vi "Analyse.vi"(0 "object in":refnum<class "StateReverse.lvclass">, 1 "NextState":string, 2 "StateAction":T1, 3 "NextStateComments":string, 5 "error in (no error)":errorcluster) -> (15 "StateTransitions":cluster{"StateTransitions":string[]}[](array[cluster]), 16 "CommentsTransitions":cluster{"StateTransitions":string[]}[](array[cluster]), 19 "error out":errorcluster)   [LabVIEW 2012, in "StateReverse.lvclass"]
uses:
  <resource>/Framework/Providers/Open_GDS/UML/StateReverse_class/StateReverse.lvclass
  <resource>/Framework/Providers/Open_GDS/UML/StateReverse_class/StateAction.ctl
  <resource>/Framework/Providers/Open_GDS/UML/ReversedEngineering/ReversedEngineering StateMachineStateInfo.ctl
  <resource>/Framework/Providers/Open_GDS/UML/StateReverse_class/StateReverse.lvclass/StateReverse.ctl
  <resource>/Framework/Providers/Open_GDS/UML/UMLEditor/UMLEditor BusyDialogAction.ctl
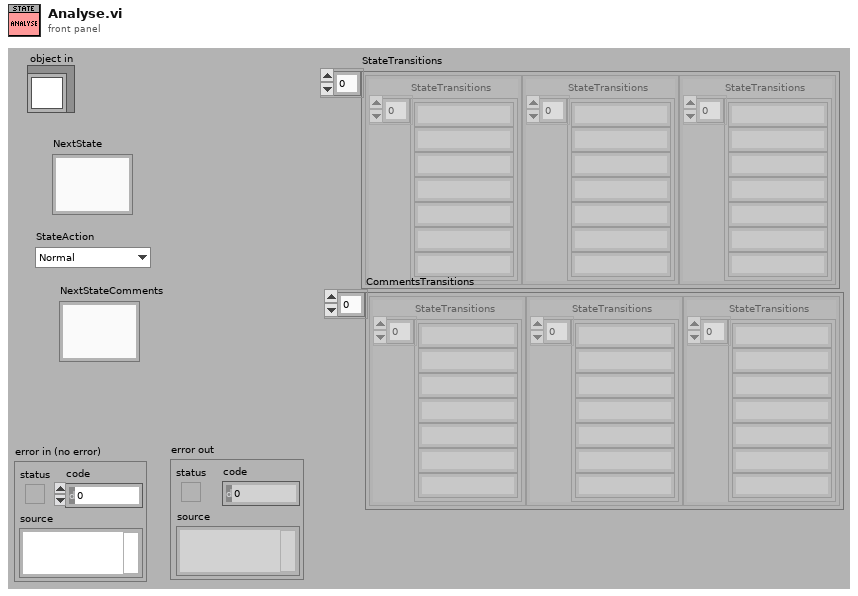
[diagram p1: front panel]
types:
  T1 = typedef "StateReverse.lvclass/StateAction.ctl" = enum16{"Normal", "AddInBeggining", "AddInEnd", "AddIfNothingInQueue"}
  T2 = typedef "ReversedEngineering StateMachineStateInfo.ctl" = cluster{"State":string, "TransitionStates":string[], "Actions":string[], "Comments":string[], "TransactionText":string[]}
  T3 = typedef "UMLEditor BusyDialogAction.ctl" = enum16{"Initialize", "Open(VIs)", "Open(i)", "Send_I-Value", "SendStatusMessage", "GetBusyDialogStatus", "Close", "Quit"}
  T4 = typedef "StateReverse.lvclass/StateDetails.ctl" = cluster{"State":string, "NextStates":T5[], "QueueUsed":bool}
  T5 = typedef "StateReverse.lvclass/NextStateAction.ctl" = cluster{"State(s)":string, "StateAction":T1, "Arg(s)":string, "Comment(s)":string}
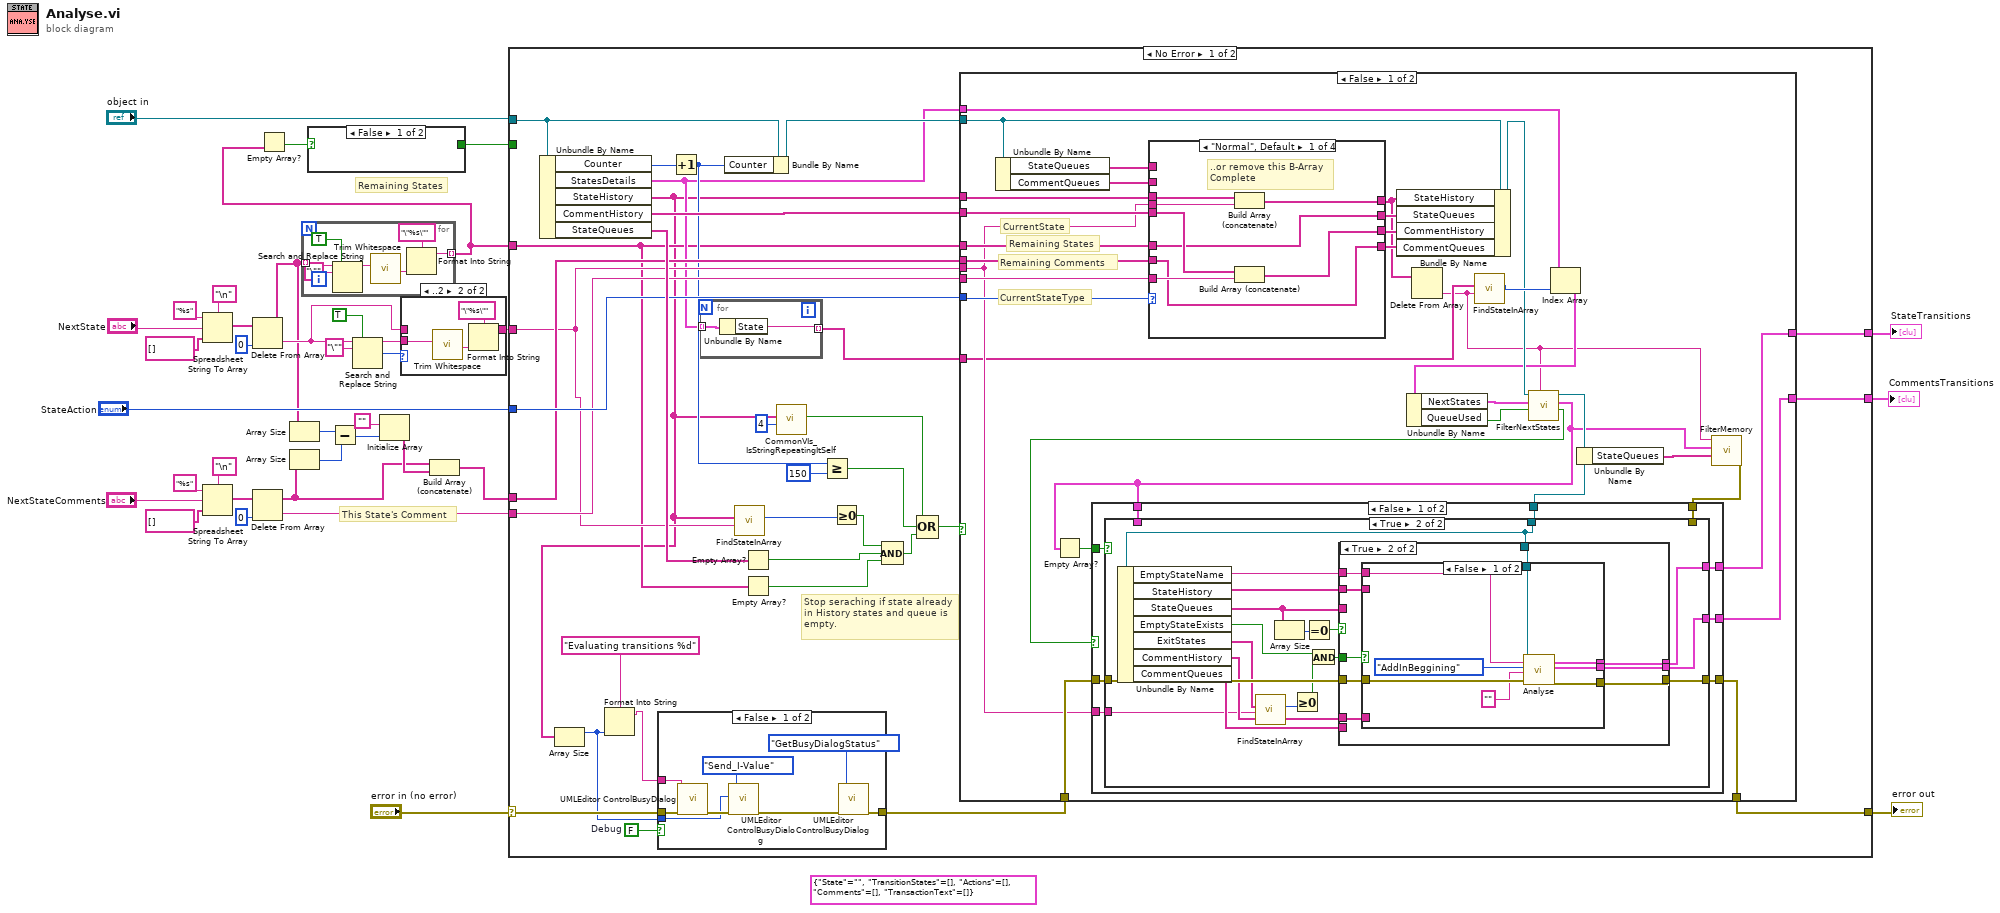
[diagram p0: block diagram]
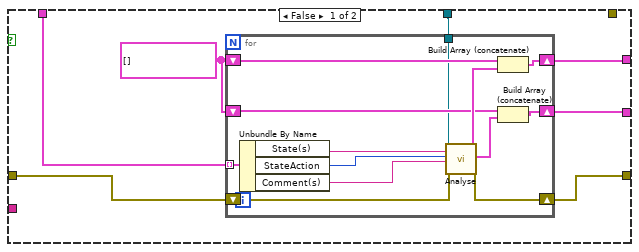
[diagram p5: hidden frame]
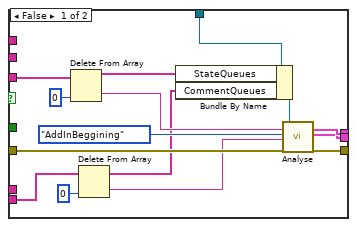
[diagram p6: hidden frame]
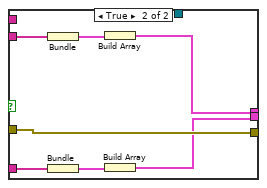
[diagram p7: hidden frame]
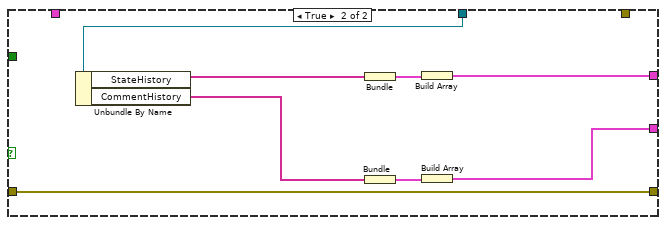
[diagram p8: hidden frame]
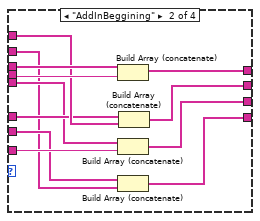
[diagram p9: hidden frame]
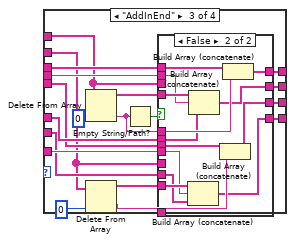
[diagram p10: hidden frame]
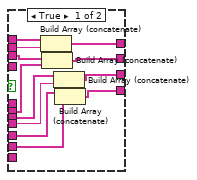
[diagram p11: hidden frame]
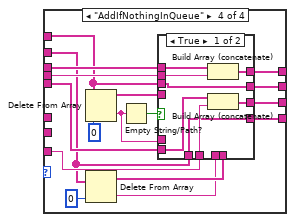
[diagram p12: hidden frame]
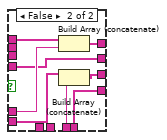
[diagram p13: hidden frame]
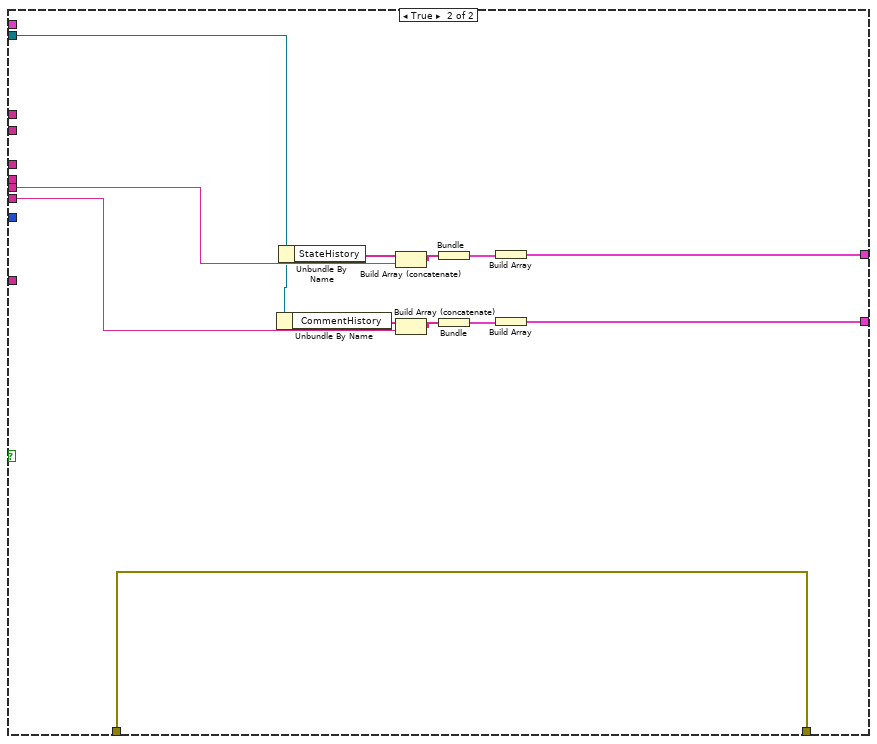
[diagram p14: hidden frame]
diagram:
  (unwired) T2 {"State"="", "TransitionStates"=[], "Actions"=[], "Comments"=[], "TransactionText"=[]} ("State")
  # "This State's Comment"
  # "Remaining States"
  n1 = Spreadsheet String To Array(delimiter (Tab)="\n", format string="%s", spreadsheet string="NextState", array type (2D Dbl)=string[] []) -> (array=w26:string[])
  n2 = Spreadsheet String To Array(delimiter (Tab)="\n", format string="%s", spreadsheet string="NextStateComments", array type (2D Dbl)=string[] []) -> (array=w18:string[])
  n3 = Delete From Array(array=w26, index=0) -> (deleted portion=w20:string, array with subset deleted=w11:string[])  [unwired: 1 in]
  n4 = Delete From Array(array=w18, index=0) -> (deleted portion=w13:string, array with subset deleted=w5:string[])  [unwired: 1 in]
  n5 = Array Size(array=w11) -> (size(s)=w10:i32)
  n6 = Array Size(array=w5) -> (size(s)=w9:i32)
  n7 = for {
    tunnel: w11 -> [w38] mode=indexing
    tunnel: [w37] -> w3 mode=indexing
    n8 = Search and Replace String(replace all?=TRUE ("replace all? (F)"), input string=w38, search string="\"") -> (result string=w41:string)  [unwired: 1 in, 7 out]
    n9 = call <vilib>:"Trim Whitespace.vi"("string"=w41) -> ("trimmed string"=w43:string)  [unwired: 1 in]
    n10 = Format Into String(format string="\"%s\"", w43) -> (resulting string=w37:string)  [unwired: 2 in, 1 out]
  }
  n11 = Empty Array?(array=w3) -> (empty?=w2:bool)
  n12 = case shown="False" w2 {
    selector: w2 -> [_ w44]
    tunnel: [_ w44] -> w1
    frame False {
    }
    frame True {
    }
  }
  n13 = Subtract(x=w10, y=w9) -> (x-y=w8:i32)
  n14 = Search and Replace String(replace all?=TRUE ("replace all? (F)"), input string=w20, search string="\"") -> (result string=w32:string, number of replacements=w21:i32)  [unwired: 1 in, 6 out]
  n15 = Initialize Array("", w8) -> (w6:string[])
  n16 = case shown="..2" w21 {
    tunnel: w32 -> [_ w49]
    tunnel: [w45 w46] -> w31
    tunnel: w20 -> [w45 _]
    frame 3.., Default {
    }
    frame ..2 {
      n17 = call <vilib>:"Trim Whitespace.vi"("string"=w49) -> ("trimmed string"=w47:string)  [unwired: 1 in]
      n18 = Format Into String(format string="\"%s\"", w47) -> (resulting string=w46:string)  [unwired: 2 in, 1 out]
    }
  }
  n19 = Build Array (concatenate)(w5, w6) -> (w4:string[])
  n20 = case shown="No Error" "error in (no error)" {
    selector: "error in (no error)" -> [w56 w330]
    tunnel: [w79 w330] -> w35
    tunnel: "object in" -> [w70 _]
    tunnel: [w80 _] -> w30
    tunnel: "StateAction" -> [w78 _]
    tunnel: w31 -> [w71 _]
    tunnel: w3 -> [w60 _]
    tunnel: w13 -> [w75 _]
    tunnel: w4 -> [w77 _]
    tunnel: [w74 _] -> w12
    tunnel: w1 -> [_ _]
    frame No Error {
      w54 = FALSE  # Debug
      # "Stop seraching if state already\nin History states and queue is\nempty."
      n21 = Unbundle By Name(w70) -> ("Counter"=w68:i32, "StatesDetails"=w61:T4[], "StateHistory"=w53:string[], "CommentHistory"=w76:string[], "StateQueues"=w82:string[])
      n22 = Array Size(array=w53) -> (size(s)=w50:i32)
      n23 = Format Into String(format string="Evaluating transitions %d", w50) -> (resulting string=w51:string)  [unwired: 2 in, 1 out]
      n24 = case shown="False" w54 {
        tunnel: w51 -> [w90 _]
        tunnel: w50 -> [w87 _]
        tunnel: w56 -> [w85 w91]
        tunnel: [w83 w91] -> w55
        frame False {
          n25 = call <resource>:"UMLEditor ControlBusyDialog.vi"("Title/StatusText"=w90, "error in (no error)"=w85) -> ("error out"=w89:errorcluster)  [unwired: 2 in, 15 out]
          n26 = call <resource>:"UMLEditor ControlBusyDialog.vi"("I-Value"=w87, "error in (no error)"=w89, "Action(SendStatusMessage)"=UMLEditor_BusyDialogAction."Send_I-Value") -> ("error out"=w84:errorcluster)  [unwired: 1 in, 15 out]
          n27 = call <resource>:"UMLEditor ControlBusyDialog.vi"("error in (no error)"=w84, "Action(SendStatusMessage)"=UMLEditor_BusyDialogAction."GetBusyDialogStatus") -> ("error out"=w83:errorcluster)  [unwired: 2 in, 15 out]
        }
        frame True {
        }
      }
      n28 = Increment(x=w68) -> (x+1=w67:i32)
      n29 = for {
        tunnel: w61 -> [w329] mode=indexing
        tunnel: [w328] -> w62 mode=indexing
        n30 = Unbundle By Name(w329) -> ("State"=w328:string)
      }
      n31 = Bundle By Name(cluster=w70, "Counter"=w67) -> (w69:refnum<class "StateReverse.lvclass">)
      n32 = call <resource>:"FindStateInArray.vi"("TransactionState"=w71, "AllCaseStates"=w53) -> ("index of element"=w73:i32)  [unwired: 9 out]
      n33 = Empty Array?(array=w82) -> (empty?=w81:bool)
      n34 = Empty Array?(array=w60) -> (empty?=w59:bool)
      n35 = call <resource>:"CommonVIs_IsStringRepeatingItSelf.vi"("Repeats(3)"=u8 4, "StateHistory"=w53) -> ("Repeating"=w58:bool)  [unwired: 9 in]
      n36 = Greater Or Equal?(x=w67, y=150) -> (x >= y?=w65:bool)
      n37 = Greater Or Equal To 0?(x=w73) -> (x >= 0?=w72:bool)
      n38 = Compound Arithmetic op=AND(w72, w81, w59) -> (w64:bool)
      n39 = Compound Arithmetic op=OR(w58, w65, w64) -> (w63:bool)
      n40 = case shown="False" w63 {
        tunnel: [w111 w325] -> w80
        tunnel: w53 -> [w123 _]
        tunnel: w71 -> [w109 w323]
        tunnel: w69 -> [w122 w318]
        tunnel: w55 -> [w121 w327]
        tunnel: [w99 w327] -> w79
        tunnel: w78 -> [w120 _]
        tunnel: w60 -> [w119 _]
        tunnel: w77 -> [w117 _]
        tunnel: w76 -> [w116 _]
        tunnel: w75 -> [w112 w317]
        tunnel: [w110 w316] -> w74
        tunnel: w62 -> [w95 _]
        tunnel: w61 -> [w106 _]
        frame False {
          # "CurrentState"
          # "CurrentStateType"
          # "Remaining Comments"
          # "Remaining States"
          n41 = Unbundle By Name(w122) -> ("StateQueues"=w118:string[], "CommentQueues"=w113:string[])
          n42 = case shown="\"Normal\", Default" w120 {
            tunnel: w123 -> [w225 w236 w256 w299]
            tunnel: w109 -> [w224 w237 w252 w295]
            tunnel: [w223 w235 w255 w298] -> w104
            tunnel: w118 -> [_ w234 w251 w294]
            tunnel: [w219 w233 w250 w293] -> w108
            tunnel: w119 -> [w219 w232 w247 _]
            tunnel: w117 -> [w218 w228 w242 _]
            tunnel: w116 -> [w222 w230 w244 w289]
            tunnel: [w221 w231 w246 w290] -> w115
            tunnel: [w218 w226 w245 w286] -> w114
            tunnel: w113 -> [_ w227 w240 w283]
            tunnel: w112 -> [w220 w229 w243 w288]
            frame "Normal", Default {
              # "..or remove this B-Array\nComplete"
              n43 = Build Array (concatenate)(w225, w224) -> (w223:string[])
              n44 = Build Array (concatenate)(w222, w220) -> (w221:string[])
            }
            frame "AddInBeggining" {
              n45 = Build Array (concatenate)(w236, w237) -> (w235:string[])
              n46 = Build Array (concatenate)(w230, w229) -> (w231:string[])
              n47 = Build Array (concatenate)(w228, w227) -> (w226:string[])
              n48 = Build Array (concatenate)(w232, w234) -> (w233:string[])
            }
            frame "AddInEnd" {
              n49 = Delete From Array(array=w251, index=0) -> (deleted portion=w249:string, array with subset deleted=w248:string[])  [unwired: 1 in]
              n50 = Delete From Array(array=w240, index=0) -> (deleted portion=w238:string, array with subset deleted=w239:string[])  [unwired: 1 in]
              n51 = Empty String/Path?(string/path=w249) -> (empty?=w253:bool)
              n52 = case shown="False" w253 {
                tunnel: w256 -> [w268 w282]
                tunnel: [w266 w281] -> w255
                tunnel: w252 -> [w267 w278]
                tunnel: w251 -> [w265 _]
                tunnel: [w264 w277] -> w250
                tunnel: w249 -> [_ w280]
                tunnel: w248 -> [_ w279]
                tunnel: w247 -> [w263 w276]
                tunnel: [w262 w275] -> w246
                tunnel: [w261 w269] -> w245
                tunnel: w244 -> [w260 w271]
                tunnel: w240 -> [w259 _]
                tunnel: w243 -> [w258 w273]
                tunnel: w242 -> [w257 w272]
                tunnel: w239 -> [_ w274]
                tunnel: w238 -> [_ w270]
                frame True {
                  n53 = Build Array (concatenate)(w268, w267) -> (w266:string[])
                  n54 = Build Array (concatenate)(w265, w263) -> (w264:string[])
                  n55 = Build Array (concatenate)(w260, w258) -> (w262:string[])
                  n56 = Build Array (concatenate)(w259, w257) -> (w261:string[])
                }
                frame False {
                  n57 = Build Array (concatenate)(w274, w273, w272) -> (w269:string[])
                  n58 = Build Array (concatenate)(w279, w278, w276) -> (w277:string[])
                  n59 = Build Array (concatenate)(w271, w270) -> (w275:string[])
                  n60 = Build Array (concatenate)(w282, w280) -> (w281:string[])
                }
              }
            }
            frame "AddIfNothingInQueue" {
              n61 = Delete From Array(array=w294, index=0) -> (deleted portion=w292:string, array with subset deleted=w291:string[])  [unwired: 1 in]
              n62 = Delete From Array(array=w283, index=0) -> (deleted portion=w284:string, array with subset deleted=w285:string[])  [unwired: 1 in]
              n63 = Empty String/Path?(string/path=w292) -> (empty?=w296:bool)
              n64 = case shown="True" w296 {
                tunnel: w299 -> [w307 w315]
                tunnel: [w304 w314] -> w298
                tunnel: w295 -> [w306 _]
                tunnel: w294 -> [w305 _]
                tunnel: [w305 w312] -> w293
                tunnel: w292 -> [_ w313]
                tunnel: w291 -> [_ w312]
                tunnel: [w303 w311] -> w290
                tunnel: w289 -> [w302 w310]
                tunnel: w288 -> [w301 _]
                tunnel: [w300 w309] -> w286
                tunnel: w285 -> [_ w309]
                tunnel: w284 -> [_ w308]
                tunnel: w283 -> [w300 _]
                frame True {
                  n65 = Build Array (concatenate)(w307, w306) -> (w304:string[])
                  n66 = Build Array (concatenate)(w302, w301) -> (w303:string[])
                }
                frame False {
                  n67 = Build Array (concatenate)(w315, w313) -> (w314:string[])
                  n68 = Build Array (concatenate)(w310, w308) -> (w311:string[])
                }
              }
            }
          }
          n69 = Bundle By Name(cluster=w122, "StateHistory"=w104, "StateQueues"=w108, "CommentHistory"=w115, "CommentQueues"=w114) -> (w102:refnum<class "StateReverse.lvclass">)
          n70 = Delete From Array(array=w104) -> (deleted portion=w94:string)  [unwired: 2 in, 1 out]
          n71 = call <resource>:"FindStateInArray.vi"("TransactionState"=w94, "AllCaseStates"=w95) -> ("index of element"=w107:i32)  [unwired: 9 out]
          n72 = Index Array(array=w106, index=w107) -> (element=w101:T4)
          n73 = Unbundle By Name(w101) -> ("NextStates"=w103:T5[], "QueueUsed"=w100:bool)
          n74 = call <resource>:"FilterNextStates.vi"("StateName"=w94, "QueueUsed(This means that the wire is connected to incoming queue elements)"=w100, "NextStates"=w103, "StateReverse in"=w102) -> ("AlreadyAnalysed"=w92:bool, "NextStatesOut"=w96:T5[], "StateReverse out"=w98:refnum<class "StateReverse.lvclass">)  [unwired: 4 in, 1 out]
          n75 = Empty Array?(array=w96) -> (empty?=w105:bool)
          n76 = Unbundle By Name(w98) -> ("StateQueues"=w97:string[])
          n77 = call <resource>:"FilterMemory.vi"("StateQueuesIn"=w97, "NextStates"=w96, "StateNameIn"=w94) -> ("error out"=w93:errorcluster)  [unwired: 5 in, 3 out]
          n78 = case shown="False" w92 {
            tunnel: w121 -> [w132 w217]
            tunnel: [w131 w211] -> w111
            tunnel: [w130 w210] -> w110
            tunnel: w109 -> [w129 _]
            tunnel: w105 -> [w128 _]
            tunnel: [w127 w217] -> w99
            tunnel: w98 -> [w126 w213]
            tunnel: w96 -> [w125 _]
            tunnel: w93 -> [w124 _]
            frame False {
              n79 = case shown="True" w128 {
                tunnel: w132 -> [w138 w170]
                tunnel: [w136 w169] -> w131
                tunnel: [w135 w168] -> w130
                tunnel: w126 -> [w134 w167]
                tunnel: [w137 w154] -> w127
                tunnel: w129 -> [_ w153]
                tunnel: w125 -> [w133 _]
                tunnel: w124 -> [_ _]
                frame False {
                  w139 = cluster{"StateTransitions":string[]}[] []
                  n80 = for {
                    tunnel: w133 -> [w152] mode=indexing
                    shift-right: [w149] -> w137
                    shift-left: w138 -> [w150]
                    shift-right: [w148] -> w136
                    shift-left: w139 -> [w147]
                    shift-right: [w144] -> w135
                    shift-left: w139 -> [w143]
                    tunnel: w134 -> [w140]
                    n81 = Unbundle By Name(w152) -> ("State(s)"=w151:string, "StateAction"=w146:T1, "Comment(s)"=w141:string)
                    n82 = call-dynamic "Analyse.vi"("object in"=w140, "NextState"=w151, "StateAction"=w146, "NextStateComments"=w141, "error in (no error)"=w150) -> ("StateTransitions"=w145:cluster{"StateTransitions":string[]}[], "CommentsTransitions"=w142:cluster{"StateTransitions":string[]}[], "error out"=w149:errorcluster)  [unwired: 12 out]
                    n83 = Build Array (concatenate)(w147, w145) -> (w148:cluster{"StateTransitions":string[]}[])
                    n84 = Build Array (concatenate)(w143, w142) -> (w144:cluster{"StateTransitions":string[]}[])
                  }
                }
                frame True {
                  n85 = Unbundle By Name(w167) -> ("EmptyStateName"=w159:string, "StateHistory"=w163:string[], "StateQueues"=w166:string[], "EmptyStateExists"=w162:bool, "ExitStates"=w156:string[], "CommentHistory"=w158:string[], "CommentQueues"=w157:string[])
                  n86 = call <resource>:"FindStateInArray.vi"("TransactionState"=w153, "AllCaseStates"=w156) -> ("index of element"=w155:i32)  [unwired: 9 out]
                  n87 = Array Size(array=w166) -> (size(s)=w165:i32)
                  n88 = Greater Or Equal To 0?(x=w155) -> (x >= 0?=w160:bool)
                  n89 = Equal To 0?(x=w165) -> (x = 0?=w164:bool)
                  n90 = And(x=w162, y=w160) -> (x .and. y?=w161:bool)
                  n91 = case shown="True" w164 {
                    tunnel: w170 -> [w185 w191]
                    tunnel: [w184 w190] -> w154
                    tunnel: [w182 w193] -> w169
                    tunnel: w167 -> [w179 w189]
                    tunnel: w166 -> [w176 _]
                    tunnel: w163 -> [_ w194]
                    tunnel: w161 -> [_ w192]
                    tunnel: w159 -> [_ w188]
                    tunnel: [w175 w187] -> w168
                    tunnel: w158 -> [_ w186]
                    tunnel: w157 -> [w171 _]
                    frame False {
                      n92 = Delete From Array(array=w176, index=0) -> (deleted portion=w181:string, array with subset deleted=w177:string[])  [unwired: 1 in]
                      n93 = Delete From Array(array=w171, index=0) -> (deleted portion=w172:string, array with subset deleted=w173:string[])  [unwired: 1 in]
                      n94 = Bundle By Name(cluster=w179, "StateQueues"=w177, "CommentQueues"=w173) -> (w178:refnum<class "StateReverse.lvclass">)
                      n95 = call-dynamic "Analyse.vi"("object in"=w178, "NextState"=w181, "StateAction"=StateAction."AddInBeggining", "NextStateComments"=w172, "error in (no error)"=w185) -> ("StateTransitions"=w182:cluster{"StateTransitions":string[]}[], "CommentsTransitions"=w175:cluster{"StateTransitions":string[]}[], "error out"=w184:errorcluster)  [unwired: 12 out]
                    }
                    frame True {
                      n96 = case shown="False" w192 {
                        tunnel: w194 -> [_ w208]
                        tunnel: [w200 w207] -> w193
                        tunnel: w191 -> [w202 w206]
                        tunnel: [w201 w206] -> w190
                        tunnel: w189 -> [w199 _]
                        tunnel: w188 -> [w198 _]
                        tunnel: [w197 w203] -> w187
                        tunnel: w186 -> [_ w204]
                        frame False {
                          n97 = call-dynamic "Analyse.vi"("object in"=w199, "NextState"=w198, "StateAction"=StateAction."AddInBeggining", "NextStateComments"="", "error in (no error)"=w202) -> ("StateTransitions"=w200:cluster{"StateTransitions":string[]}[], "CommentsTransitions"=w197:cluster{"StateTransitions":string[]}[], "error out"=w201:errorcluster)  [unwired: 12 out]
                        }
                        frame True {
                          n98 = Bundle("StateHistory"=w208) -> (w209:cluster{"StateHistory":string[]})  [unwired: 1 in]
                          n99 = Bundle("CommentHistory"=w204) -> (w205:cluster{"CommentHistory":string[]})  [unwired: 1 in]
                          n100 = Build Array(w209) -> (w207:cluster{"StateHistory":string[]}[])
                          n101 = Build Array(w205) -> (w203:cluster{"CommentHistory":string[]}[])
                        }
                      }
                    }
                  }
                }
              }
            }
            frame True {
              n102 = Unbundle By Name(w213) -> ("StateHistory"=w214:string[], "CommentHistory"=w212:string[])
              n103 = Bundle("StateHistory"=w214) -> (w216:cluster{"StateHistory":string[]})  [unwired: 1 in]
              n104 = Bundle("CommentHistory"=w212) -> (w215:cluster{"CommentHistory":string[]})  [unwired: 1 in]
              n105 = Build Array(w216) -> (w211:cluster{"StateHistory":string[]}[])
              n106 = Build Array(w215) -> (w210:cluster{"CommentHistory":string[]}[])
            }
          }
        }
        frame True {
          n107 = Unbundle By Name(w318) -> ("CommentHistory"=w320:string[])
          n108 = Unbundle By Name(w318) -> ("StateHistory"=w324:string[])
          n109 = Build Array (concatenate)(w324, w323) -> (w322:string[])
          n110 = Build Array (concatenate)(w320, w317) -> (w321:string[])
          n111 = Bundle(w322) -> (w326:cluster{string[]})  [unwired: 1 in]
          n112 = Bundle(w321) -> (w319:cluster{string[]})  [unwired: 1 in]
          n113 = Build Array(w326) -> (w325:cluster{string[]}[])
          n114 = Build Array(w319) -> (w316:cluster{string[]}[])
        }
      }
    }
    frame Error {
    }
  }
  "error out" <- w35
  "StateTransitions" <- w30
  "CommentsTransitions" <- w12
